vi "Maquette - v1.4 - final.vi"() -> ()   [LabVIEW 2019]
uses:
  <vilib>/Platform/TimedLoop/XDataNode/timing_clust.ctl
  <vilib>/Platform/TimedLoop/XDataNode/nitl_modes.ctl
  <vilib>/Platform/TimedLoop/XDataNode/wakeup.ctl
  <vilib>/Platform/TimedLoop/XDataNode/XDataNode.xnode
  <vilib>/Platform/TimedLoop/XDataNode/XDNodeRunTimeDep.lvlib
panel:
  out "Porte":u16(ring)
  in  "Servomoteur":bool
  in  "Présence":bool
  out "Lampe plafond":bool
  out "Radiateur":bool
  out "Ventilateur":bool
  in  "Température":dbl(slide) min=0.0 max=40.0 step=1.0 scale=0.0..40.0
  in  "stop":bool
  # "STAYLAZY"
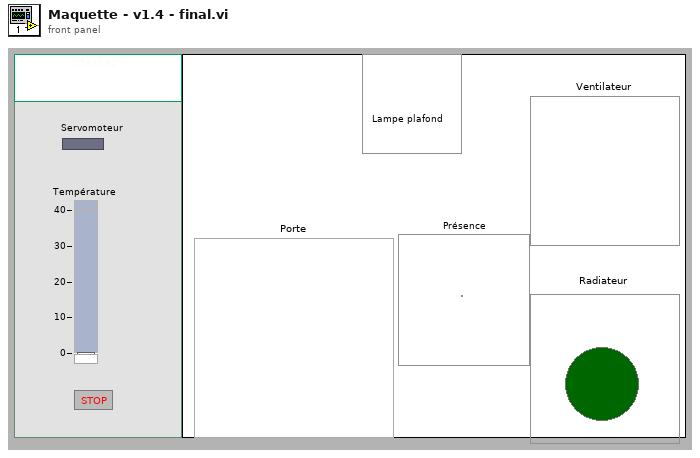
[diagram p1: front panel]
types:
  T1 = typedef "XDNodeRunTimeDep.lvlib/timing_clust.ctl" = cluster{"Expected End [f-1]":u64, "Actual End [f-1]":u64, "Finished Late? [f-1]":bool, "Expected End [i-1]":u64, "Actual End [i-1]":u64, "Finished Late? [i-1]":bool, "Expected Start [i]":u64, "Actual Start [i]":u64, "Expected Start [f]":u64, "Actual Start [f]":u64, "Source Name":string, "Structure Name":string, "Period":i64, "Deadline":i64, "Offset":i64, "Start":i64, "Priority":i32, "Timeout":i32, "Mode":T2, "Wakeup Reason":T3, "Error":errorcluster, "Source Type":string, "Secondary Source Type":string, "Global End Time":u64, "Global Start Time":u64, "Frame Duration":u64, "Iteration Duration":u64, "Assigned CPU":i32, "I/O Scan Engine Mode":u32}
  T2 = typedef "XDNodeRunTimeDep.lvlib/nitl_modes.ctl" = enum32{"No Change", "Process missed periods, maintain original phase", "Discard missed periods, maintain original phase", "Process missed periods, ignore original phase", "Discard missed periods, ignore original phase"}
  T3 = typedef "XDNodeRunTimeDep.lvlib/wakeup.ctl" = enum32{"Normal", "Aborted", "Asynchronous wakeup", "Timing source error", "Timed loop error", "Timeout"}
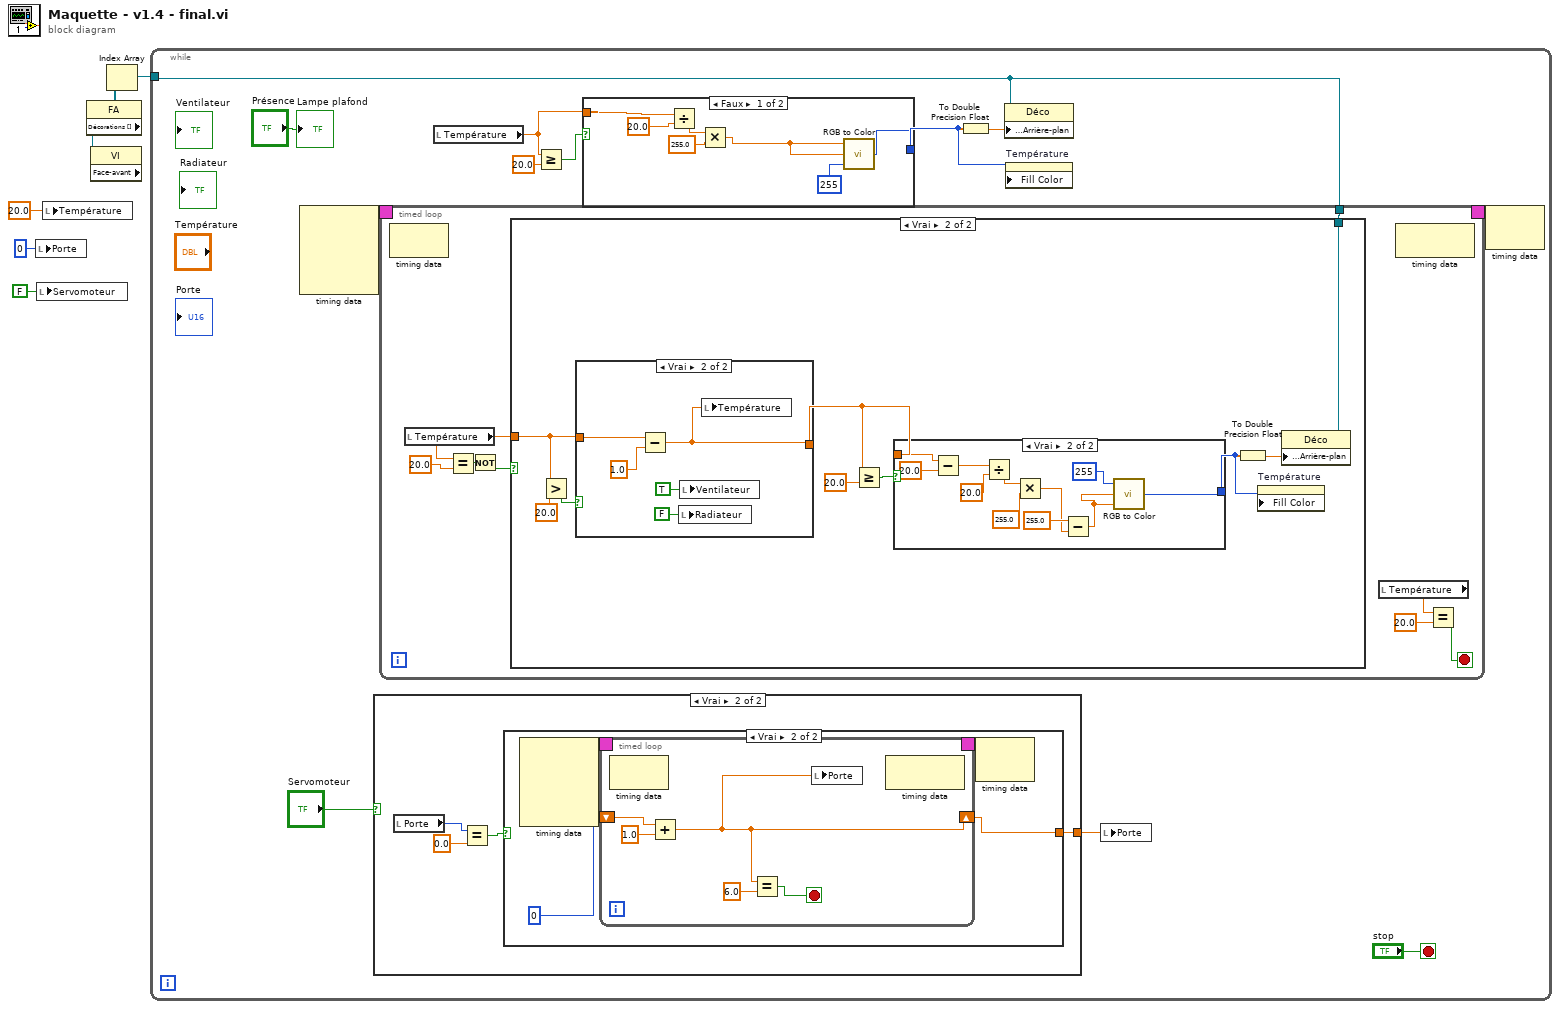
[diagram p0: block diagram]
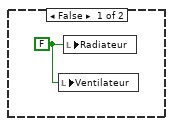
[diagram p2: hidden frame]
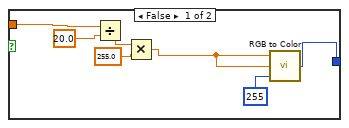
[diagram p3: hidden frame]
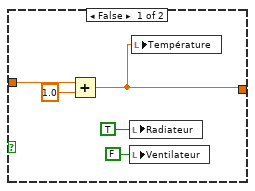
[diagram p4: hidden frame]
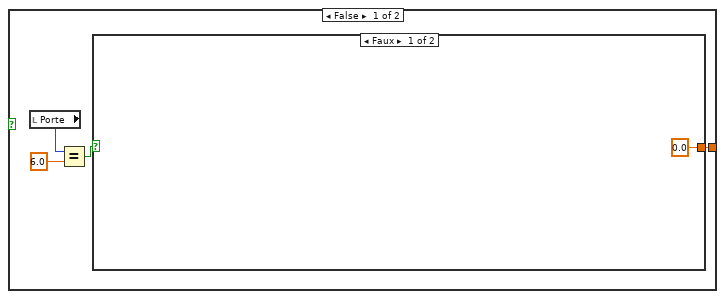
[diagram p5: hidden frame]
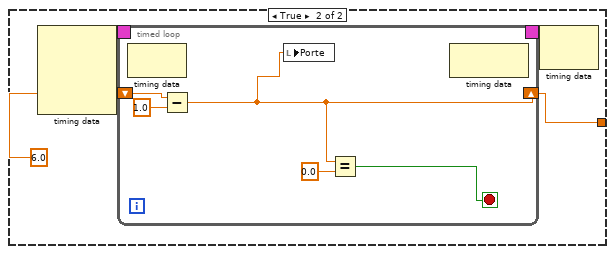
[diagram p6: hidden frame]
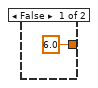
[diagram p7: hidden frame]
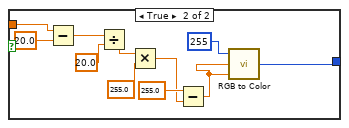
[diagram p8: hidden frame]
diagram:
  n1 = local write "Porte"(u16 0 ("Porte")) -> ()
  n2 = local write "Servomoteur"(FALSE ("Servomoteur")) -> ()
  n3 = local write "Température"(20.0 ("Thermomètre")) -> ()
  n4 = property class="VI"() -> ("Face-avant"=w6:refnum<vi>)  [unwired: 2 in, 2 out]
  n5 = property class="FA"(reference=w6) -> ("Décorations []"=w5:refnum<vi>[])  [unwired: 1 in, 2 out]
  n6 = Index Array(array=w5) -> (element=w4:refnum<vi>)  [unwired: 1 in]
  n7 = while {
    tunnel: w4 -> [w12]
    stop <- "stop" stop-if-true
    n8 = node-c288() -> (w8:T1)  [unwired: 4 in]
    n9 = case shown="Vrai" "Servomoteur" {
      tunnel: [w69 w87] -> w9
      frame False {
        n10 = local read "Porte"() -> (w71:u16)
        n11 = Equal?(x=w71, y=6.0) -> (x = y?=w70:bool)
        n12 = case shown="Faux" w70 {
          tunnel: [0.0 ("x") w74] -> w69
          frame False {
          }
          frame True {
            n13 = node-c288() -> (w77:T1)  [unwired: 4 in]
            n14 = timed-loop {
              shift-right: [w78] -> w74
              shift-left: 6.0 ("x") -> [w80]
              timing: w77 -> [_]
              timing-out: [_] -> w76
              stop <- w79 stop-if-true
              n15 = node-c288() -> ()  [unwired: 1 in, 1 out]
              n16 = Subtract(x=w80, y=1.0) -> (x-y=w78:dbl)
              n17 = local write "Porte"(w78) -> ()
              n18 = Equal?(x=w78, y=0.0) -> (x = y?=w79:bool)
              n19 = node-c288() -> ()  [unwired: 1 in, 1 out]
            }
            n20 = node-c288(w76) -> ()  [unwired: 1 out]
          }
        }
      }
      frame True {
        n21 = local read "Porte"() -> (w90:u16)
        n22 = Equal?(x=w90, y=0.0) -> (x = y?=w88:bool)
        n23 = case shown="Vrai" w88 {
          tunnel: [6.0 ("Porte") w92] -> w87
          frame False {
          }
          frame True {
            n24 = node-c288() -> (w95:T1)  [unwired: 4 in]
            n25 = timed-loop {
              shift-right: [w96] -> w92
              shift-left: u16 0 ("Porte") -> [w99]
              timing: w95 -> [_]
              timing-out: [_] -> w94
              stop <- w98 stop-if-true
              n26 = node-c288() -> ()  [unwired: 1 in, 1 out]
              n27 = Add(x=w99, y=1.0) -> (x+y=w96:dbl)
              n28 = Equal?(x=w96, y=6.0) -> (x = y?=w98:bool)
              n29 = local write "Porte"(w96) -> ()
              n30 = node-c288() -> ()  [unwired: 1 in, 1 out]
            }
            n31 = node-c288(w94) -> ()  [unwired: 1 out]
          }
        }
      }
    }
    n32 = timed-loop {
      timing: w8 -> [_]
      timing-out: [_] -> w7
      tunnel: w12 -> [w22]
      stop <- w21 stop-if-true
      n33 = node-c288() -> ()  [unwired: 1 in, 1 out]
      n34 = local read "Température"() -> (w26:dbl)
      n35 = Equal?(x=w26, y=20.0) -> (x = y?=w23:bool)
      n36 = Not(x=w23) -> (.not. x?=w24:bool)
      n37 = case shown="Vrai" w24 {
        tunnel: w26 -> [_ w36]
        tunnel: w22 -> [_ w35]
        frame False {
          w27 = FALSE ("Thermostat")
          n38 = local write "Ventilateur"(w27) -> ()
          n39 = local write "Radiateur"(w27) -> ()
        }
        frame True {
          n40 = Greater?(x=w36, y=20.0) -> (0:w33:bool)
          n41 = case shown="Vrai" w33 {
            tunnel: w36 -> [w59 w64]
            tunnel: [w56 w62] -> w29
            frame False {
              n42 = Add(x=w59, y=1.0) -> (x+y=w56:dbl)
              n43 = local write "Radiateur"(TRUE ("Thermostat")) -> ()
              n44 = local write "Ventilateur"(FALSE ("Ventilateur")) -> ()
              n45 = local write "Température"(w56) -> ()
            }
            frame True {
              n46 = Subtract(x=w64, y=1.0) -> (x-y=w62:dbl)
              n47 = local write "Radiateur"(FALSE ("Radiateur")) -> ()
              n48 = local write "Ventilateur"(TRUE ("Ventilateur")) -> ()
              n49 = local write "Température"(w62) -> ()
            }
          }
          n50 = Greater Or Equal?(x=w29, y=20.0) -> (x >= y?=w31:bool)
          n51 = case shown="Vrai" w31 {
            tunnel: w29 -> [w38 w53]
            tunnel: [w40 w44] -> w28
            frame False {
              n52 = Divide(x=w38, y=20.0) -> (x/y=w41:dbl)
              n53 = Multiply(x=w41, y=255.0) -> (x*y=w37:dbl)
              n54 = call <vilib>:"RGB to Color.vi"("B"=u8 255 ("R"), "G"=w37, "R"=w37) -> ("Color"=w40:u32)
            }
            frame True {
              n55 = Subtract(x=w53, y=20.0) -> (x-y=w52:dbl)
              n56 = Divide(x=w52, y=20.0) -> (x/y=w49:dbl)
              n57 = Multiply(x=w49, y=255.0) -> (x*y=w46:dbl)
              n58 = Subtract(x=255.0, y=w46) -> (x-y=w45:dbl)
              n59 = call <vilib>:"RGB to Color.vi"("B"=w45, "G"=w45, "R"=u8 255) -> ("Color"=w44:u32)
            }
          }
          n60 = To Double Precision Float(number=w28) -> (double precision float=w30:dbl)
          n61 = property on="Température" class="Gliss (strict)"("Fill Color"=w28) -> ()  [unwired: 2 in, 2 out]
          n62 = property class="Déco"(reference=w35, "Couleurs:Arrière-plan"=w30) -> ()  [unwired: 1 in, 2 out]
        }
      }
      n63 = local read "Température"() -> (w20:dbl)
      n64 = node-c288() -> ()  [unwired: 1 in, 1 out]
      n65 = Equal?(x=w20, y=20.0) -> (x = y?=w21:bool)
    }
    n66 = local read "Température"() -> (w13:dbl)
    n67 = Greater Or Equal?(x=w13, y=20.0) -> (x >= y?=w16:bool)
    n68 = case shown="Faux" w16 {
      tunnel: w13 -> [w106 w121]
      tunnel: [w108 w112] -> w14
      frame False {
        n69 = Divide(x=w106, y=20.0) -> (x/y=w109:dbl)
        n70 = Multiply(x=w109, y=255.0) -> (x*y=w105:dbl)
        n71 = call <vilib>:"RGB to Color.vi"("B"=u8 255 ("R"), "G"=w105, "R"=w105) -> ("Color"=w108:u32)
      }
      frame True {
        n72 = Subtract(x=w121, y=20.0) -> (x-y=w120:dbl)
        n73 = Divide(x=w120, y=20.0) -> (x/y=w117:dbl)
        n74 = Multiply(x=w117, y=255.0) -> (x*y=w114:dbl)
        n75 = Subtract(x=255.0, y=w114) -> (x-y=w113:dbl)
        n76 = call <vilib>:"RGB to Color.vi"("B"=w113, "G"=w113, "R"=u8 255) -> ("Color"=w112:u32)
      }
    }
    n77 = To Double Precision Float(number=w14) -> (double precision float=w15:dbl)
    n78 = property class="Déco"(reference=w12, "Couleurs:Arrière-plan"=w15) -> ()  [unwired: 1 in, 2 out]
    n79 = property on="Température" class="Gliss (strict)"("Fill Color"=w14) -> ()  [unwired: 2 in, 2 out]
    n80 = local write "Porte"(w9) -> ()
    n81 = node-c288(w7) -> ()  [unwired: 1 out]
    "Lampe plafond" <- "Présence"
  }
